vi "Set Traverse Classes.vi"(6 "Traverse classes? [F]":bool, 8 "error in (no error)":errorcluster, 11 "Registry Ctrl Ref Accessor in":refnum<class "Registry Ctrl Ref Accessor.lvclass">) -> (0 "error out":errorcluster, 3 "Registry Ctrl Ref Accessor out":refnum<class "Registry Ctrl Ref Accessor.lvclass">)   [LabVIEW 2013, in "Registry Ctrl Ref Accessor.lvclass"]
doc: "Copyright 2018, Carya Automatisering, Wiebe Walstra."
uses:
  Registry Ctrl Ref Accessor.lvclass
  Registry Ctrl Ref Accessor.lvclass/Registry Ctrl Ref Accessor.ctl
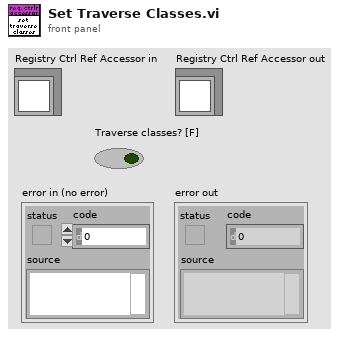
[diagram p1: front panel]
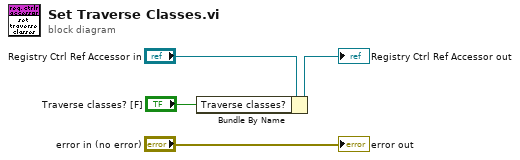
[diagram p0: block diagram]
diagram:
  n1 = Bundle By Name(cluster="Registry Ctrl Ref Accessor in", "Traverse classes?"="Traverse classes? [F]") -> (→"Registry Ctrl Ref Accessor out":refnum<class "Registry Ctrl Ref Accessor.lvclass">)
  "error out" <- "error in (no error)"
